vi "S30c_dll F31.vi"(4 "error in":errorcluster, 5 "Nr.":u8, 6 "Coefficient":sgl format="%_6f", 7 "Dev Addr":u8=250) -> (0 "error out":errorcluster)   [LabVIEW 2014, in "K_S30c_dll.lvlib"]
uses:
  K_S30c_dll.lvlib
  s30c.dll
panel:
  # "Function31: Write coefficient  \n\nusing s30c.dll\nKeller AG für Druckmesstechnik, 29.5.08 b.v."
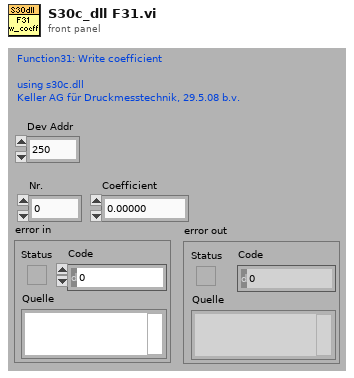
[diagram p1: front panel]
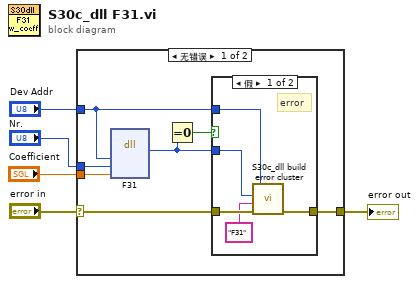
[diagram p0: block diagram]
diagram:
  n1 = case shown="无错误" "error in" {
    selector: "error in" -> [w10 w19]
    tunnel: [w11 w19] -> w3
    tunnel: "Dev Addr" -> [w9 _]
    tunnel: "Nr." -> [w7 _]
    tunnel: "Coefficient" -> [w6 _]
    frame No Error {
      n2 = dll-call lib="PTH2Labs EworkSINOPEC北控自动相渗software2.08.5_dlls30c.dll" fn="F31"("DevAddr"=w9, "Coeff No"=w7, "Coeff"=w6) -> (w8:i16)  [unwired: 6 in, 2 out]
      n3 = Equal To 0?(x=w8) -> (x = 0?=w12:bool)
      n4 = case shown="假" w12 {
        tunnel: w10 -> [w17 w18]
        tunnel: [w16 w18] -> w11
        tunnel: w9 -> [w14 _]
        tunnel: w8 -> [w13 _]
        frame False {
          # "error"
          n5 = call "S30c_dll build error cluster.vi"("error in"=w17, "error Text"="F31", "error code"=w13, "Dev Addr"=w14) -> ("error out"=w16:errorcluster)  [unwired: 3 in]
        }
        frame True {
        }
      }
    }
    frame Error {
    }
  }
  "error out" <- w3
